vi "Actor Loop.vi"(11 "Actor in":refnum<class "Actor.lvclass">) -> (3 "Actor out":refnum<class "Actor.lvclass">)   [LabVIEW 2021, in "LVCAM.lvlib" / "Actor.lvclass"]
uses:
  Actor.lvclass
  Msg Strategy/Msg Strategy.lvclass
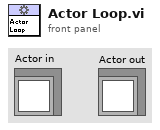
[diagram p1: front panel]
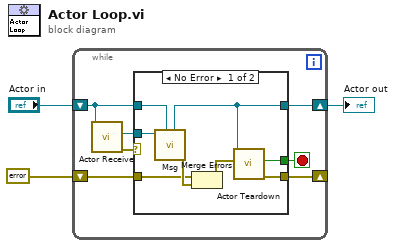
[diagram p0: block diagram]
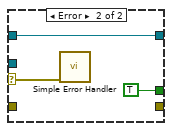
[diagram p2: hidden frame]
diagram:
  n1 = while {
    shift-right: [w10] -> w1
    shift-left: "Actor in" -> [w4]
    shift-right: [w6] -> _
    shift-left: errorcluster {"status"=FALSE, "code"=0, "source"=""} ("error IO") -> [w5]
    stop <- w8 stop-if-true
    n2 = call-dynamic "Actor Receive.vi"("Actor in"=w4) -> ("error out"=w7:errorcluster, "Msg"=w9:refnum<class "Msg Strategy.lvclass">)  [unwired: 9 in]
    n3 = case shown="No Error" w7 {
      selector: w7 -> [_ w19]
      tunnel: [w11 w21] -> w10
      tunnel: w9 -> [w18 _]
      tunnel: [w16 TRUE ("Destroyed Self?")] -> w8
      tunnel: w4 -> [w17 w21]
      tunnel: [w15 _] -> w6
      tunnel: w5 -> [w12 _]
      frame No Error {
        n4 = call-dynamic "Msg.vi"("Actor in"=w17, "Msg Strategy in"=w18) -> ("error out"=w13:errorcluster, "Actor out"=w11:refnum<class "Actor.lvclass">)  [unwired: 8 in]
        n5 = Merge Errors(w12, w13) -> (w14:errorcluster)
        n6 = call-dynamic "Actor Teardown.vi"("Error"=w14, "Actor in"=w11) -> ("error out"=w15:errorcluster, "Teardown?"=w16:bool)  [unwired: 8 in]
      }
      frame Error {
        n7 = call <vilib>:"Simple Error Handler.vi"("error in (no error)"=w19) -> ()  [unwired: 4 in, 5 out]
      }
    }
  }
  "Actor out" <- w1
